vi "ConfigAll.vi"(8 "error in (no error)":errorcluster, 11 "Stand in":refnum<class "Stand.lvclass">) -> (0 "error out":errorcluster, 1 "logger out":refnum<class "Logger.lvclass">, 2 "ModbusSp out":refnum<class "ModbusSp.lvclass">, 3 "Stand out":refnum<class "Stand.lvclass">, 4 "FPGA_Interface":refnum<class "FPGA_Interface.lvclass">)   [LabVIEW 2019, in "Stand.lvclass"]
uses:
  Stand.lvclass
  C:/Users/H4001/Documents/GitHub/H4000/src/Proccess_class/Proccess.lvclass
  Logger_class/Logger.lvclass
  Modbus_class/ModbusSp.lvclass
  FPGA_Interface_class/FPGA_Interface.lvclass
  Database_Postgress_class/Database_Postgress.lvclass
  C:/Users/H4001/Documents/GitHub/H4000/src/DatabaseInterface_class/DatabaseInterface.lvclass
  Database_Postgress_class/Connection Info.ctl
  ConfigJSON_class/ConfigJSON.lvclass
  C:/Users/H4001/Documents/GitHub/H4000/src/ConfigInterface_class/ConfigInterface.lvclass
  MessageAMC_class/MessageAMC.lvclass
  C:/Users/H4001/Documents/GitHub/H4000/src/MessageInterface_class/MessageInterface.lvclass
  TypeDef/State.ctl
  FPGA_Concrete_class/FPGA_Concrete.lvclass
  C:/Users/H4001/Documents/GitHub/H4000/src/FPGA_Interface_class/FPGA_Interface.lvclass
  ConfigJSON_class/ConfigJSON.lvclass/ConfigJSON.ctl
  Stand.lvclass/Stand.ctl
  d5dec137-e01f-4e74-a2ba-f6c6d38a38a1.vi
  Proccess_class/Proccess.lvclass
  DatabaseInterface_class/DatabaseInterface.lvclass
  FPGA_Mock_class/FPGA_Mock.lvclass
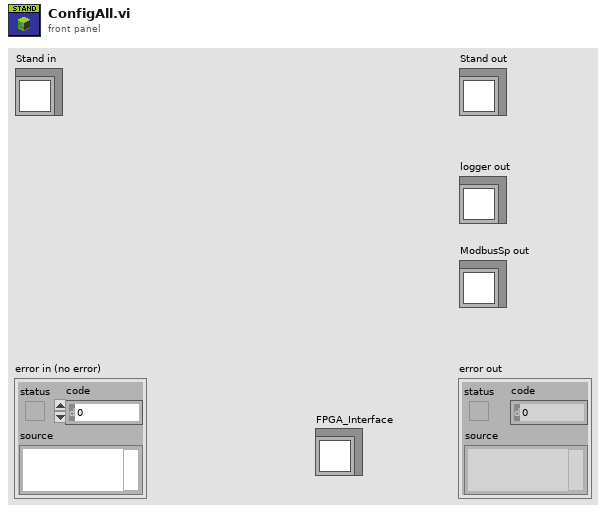
[diagram p1: front panel]
types:
  T1 = typedef "State.ctl" = enum16{"INIT", "IDLE", "CHANNEL_TESTING", "OIL_FILLING", "PREPARE_TO_HI_PRESS", "HI_PRESSURE", "ALARM", "HI PRESSURE TEST"}
  T2 = typedef "DatabaseInterface.lvclass/Connection Info.ctl" = cluster{"IP_Address":string, "Port":u16, "Timeout":i32, "User":string, "Password":string, "Database":string}
  T3 = typedef "Devices.ctl" = cluster{"AIs":refnum<class "Sig_AI.lvclass">[], "DIs":refnum<class "Sig_DI_Simple.lvclass">[], "DOs":refnum<class "Sig_DO_Simple.lvclass">[], "PUMPs":refnum<class "Engine_1DI_2DO.lvclass">[], "AOs":refnum<class "Sig_AO.lvclass">[], "MB_ENGINE 1":refnum<class "MB_ENGINE.lvclass">, "ValveModbus 1":refnum<class "ValveModbus.lvclass">}
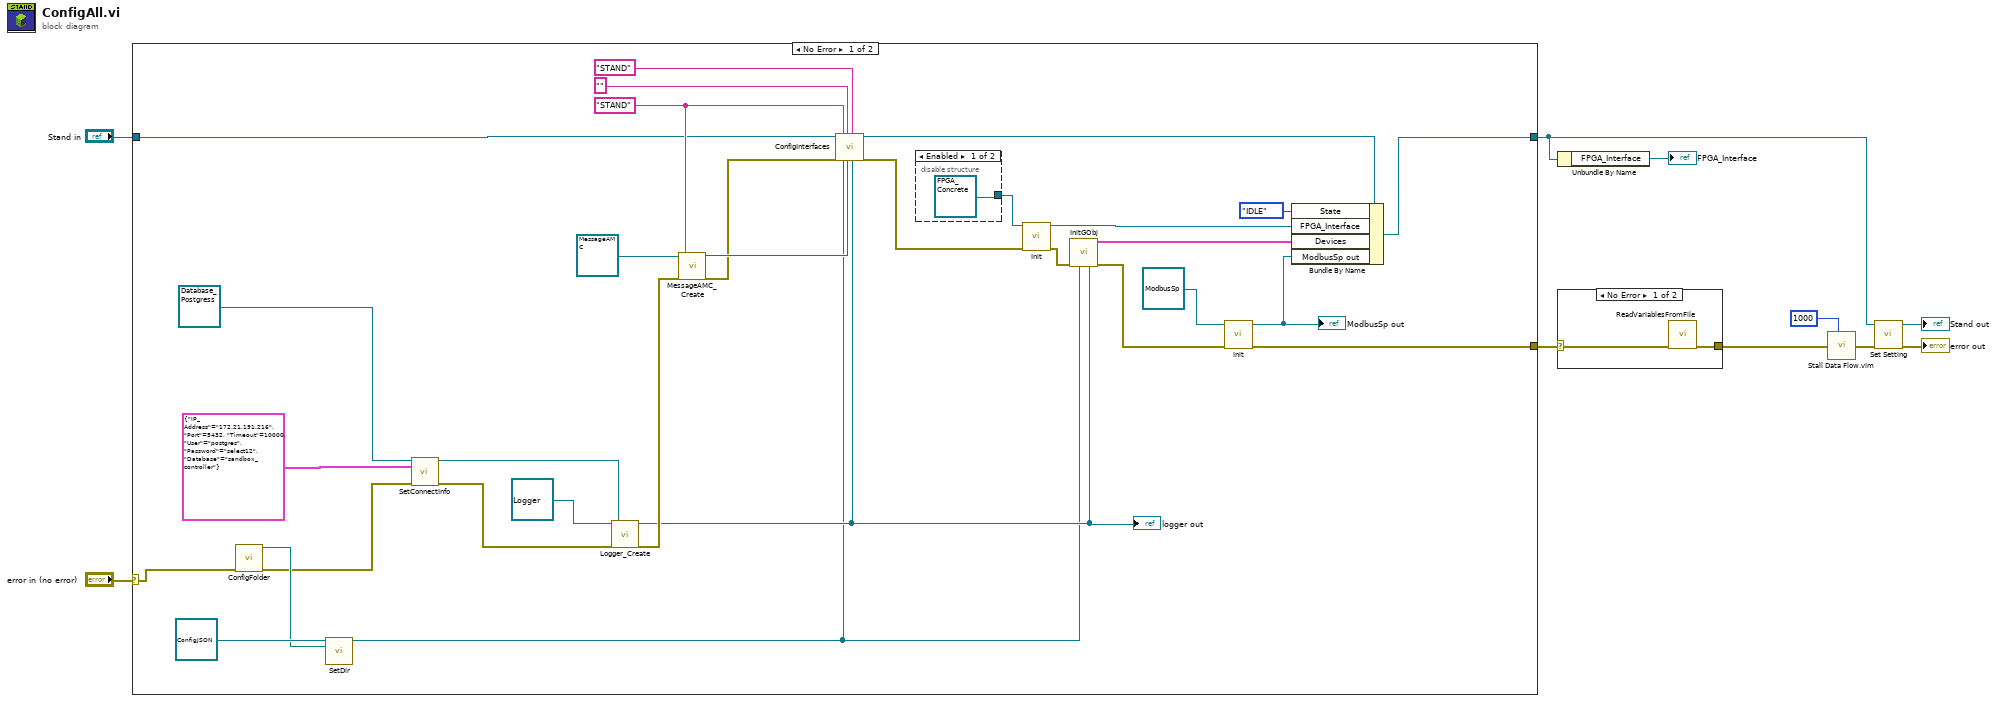
[diagram p0: block diagram]
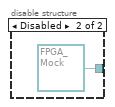
[diagram p3: hidden frame]
diagram:
  n1 = case shown="No Error" "error in (no error)" {
    selector: "error in (no error)" -> [w14 w45]
    tunnel: [w21 w45] -> w7
    tunnel: [w27 w44] -> w3
    tunnel: "Stand in" -> [w29 w44]
    frame No Error {
      w32 = "STAND" ("Name")
      n2 = call "ConfigFolder.vi"("error in (no error)"=w14) -> ("dup path"=w15:path, "error out"=w13:errorcluster)  [unwired: 13 in]
      n3 = call "SetDir.vi"("reference in"=refnum<class "ConfigJSON.lvclass"> refnum ("ConfigJSON"), "Config Dir"=w15) -> ("JSON"=w12:refnum<class "ConfigJSON.lvclass">)  [unwired: 13 in]
      n4 = call-dynamic "SetConnectInfo.vi"("reference in"=refnum<class "Database_Postgress.lvclass"> refnum, "Connection Info"=T2 {"IP_Address"="172.21.191.216", "Port"=5432, "Timeout"=10000, "User"="postgres", "Password"="select12", "Database"="sandbox_controller"}, "error in (no error)"=w13) -> ("reference out"=w36:refnum<class "Database_Postgress.lvclass">, "error out"=w35:errorcluster)  [unwired: 11 in]
      n5 = call "Logger_Create.vi"("reference in"=refnum<class "Logger.lvclass"> refnum, "error in (no error)"=w35, "DatabaseInterface"=w36) -> ("reference out"=w26:refnum<class "Logger.lvclass">, "error out"=w31:errorcluster)  [unwired: 15 in]
      "logger out" <- w26
      n6 = call "MessageAMC_Create.vi"("reference in"=refnum<class "MessageAMC.lvclass"> refnum ("MessageAMC"), "error in (no error)"=w31, "message queue name"=w32) -> ("amc"=w33:refnum<class "MessageAMC.lvclass">, "error out"=w30:errorcluster)  [unwired: 15 in]
      n7 = call "ConfigInterfaces.vi"("reference in"=w29, "error in (no error)"=w30, "Name"=w32, "ConfigInterface"=w12, "ParentName"="", "MessageInterface"=w33, "Description"="STAND", "Logger"=w26) -> ("reference out"=w28:refnum<class "Stand.lvclass">, "error out"=w17:errorcluster)  [unwired: 10 in]
      n8 = disable-structure shown="Enabled" {
        disable-tunnel: [refnum<class "FPGA_Concrete.lvclass"> refnum ("reference in") refnum<class "FPGA_Mock.lvclass"> refnum ("FPGA_Sim")] -> w19
        frame Enabled {
        }
        frame Disabled {
        }
      }
      n9 = call-dynamic "Init.vi"("reference in"=w19, "error in (no error)"=w17) -> ("reference out"=w20:refnum<class "FPGA_Concrete.lvclass">, "error out"=w18:errorcluster)  [unwired: 12 in]
      n10 = call "InitGObj.vi"("error in"=w18, "ConfigInterface"=w12, "Logger"=w26) -> ("Devices"=w25:T3, "error out"=w23:errorcluster)  [unwired: 11 in]
      n11 = call "Init.vi"("error in (no error)"=w23, "ModbusSp in"=refnum<class "ModbusSp.lvclass"> refnum) -> ("error out"=w21:errorcluster, "ModbusSp out"=w22:refnum<class "ModbusSp.lvclass">)  [unwired: 8 in]
      "ModbusSp out" <- w22
      n12 = Bundle By Name(cluster=w28, "State"=State."IDLE", "FPGA_Interface"=w20, "Devices"=w25, "ModbusSp out"=w22) -> (w27:refnum<class "Stand.lvclass">)
    }
    frame Error {
    }
  }
  n13 = Unbundle By Name(w3) -> ("FPGA_Interface"=→"FPGA_Interface":refnum<class "FPGA_Interface.lvclass">)
  n14 = case shown="No Error" w7 {
    selector: w7 -> [w46 w48]
    tunnel: [w47 w48] -> w6
    frame No Error {
      n15 = call "ReadVariablesFromFile.vi"("error in (no error)"=w46) -> ("error out"=w47:errorcluster)  [unwired: 14 in]
    }
    frame Error {
    }
  }
  n16 = call "Stall Data Flow.vim"("value in"=w6, "milliseconds to wait"=u32 1000) -> ("value out"=w2:errorcluster)  [unwired: 1 out]
  n17 = call "Set Setting.vi"("error in (no error)"=w2, "Stand in"=w3) -> ("error out"=→"error out":errorcluster, "Stand out"=→"Stand out":refnum<class "Stand.lvclass">)  [unwired: 8 in]
